vi "Read Message (sent).vi"(8 "error in (no error)":errorcluster, 11 "RemoteControl in":refnum<class "RemoteControl.lvclass">) -> (0 "error out":errorcluster, 1 "Data (Sent)":variant, 2 "Command (Sent)":string, 3 "RemoteControl out":refnum<class "RemoteControl.lvclass">, 4 "ID (Sent)":string)   [LabVIEW 2019, in "RemoteControl.lvclass"]
uses:
  RemoteControl.lvclass
  RemoteControl.lvclass/RemoteControl.ctl
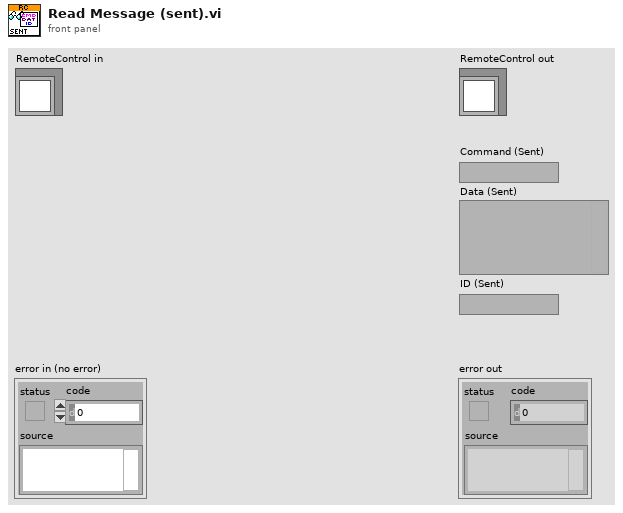
[diagram p1: front panel]
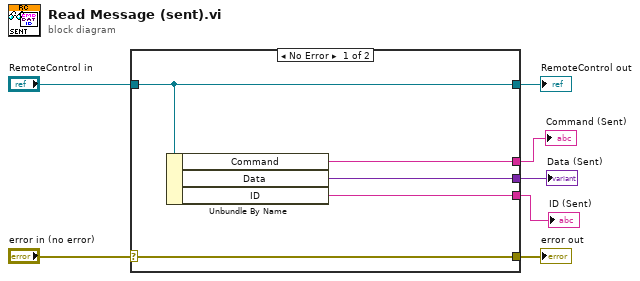
[diagram p0: block diagram]
diagram:
  n1 = case shown="No Error" "error in (no error)" {
    selector: "error in (no error)" -> [w12 w13]
    tunnel: [w12 w13] -> w6
    tunnel: [w11 w14] -> w4
    tunnel: "RemoteControl in" -> [w11 w14]
    tunnel: [w10 _] -> w3
    tunnel: [w9 _] -> w2
    tunnel: [w8 _] -> w1
    frame No Error {
      n2 = Unbundle By Name(w11) -> ("Command"=w10:string, "Data"=w9:variant, "ID"=w8:string)
    }
    frame Error {
    }
  }
  "error out" <- w6
  "RemoteControl out" <- w4
  "ID (Sent)" <- w1
  "Command (Sent)" <- w3
  "Data (Sent)" <- w2
